vi "Configure Over Voltage Limit.vi"(8 "error in (no error)":errorcluster, 10 "Over Voltage Setting":T1, 11 "BK-Precision in":refnum<class "BK-Precision.lvclass">) -> (0 "error out":errorcluster, 3 "BK-Precision out":refnum<class "BK-Precision.lvclass">)   [LabVIEW 2021, in "DC PWS.lvlib" / "BK-Precision.lvclass"]
uses:
  BK-Precision.lvclass
  BK-Precision.lvclass/BK-Precision.ctl
  <instrlib>/BK Precision 911X Series/BK Precision 911X Series.lvlib
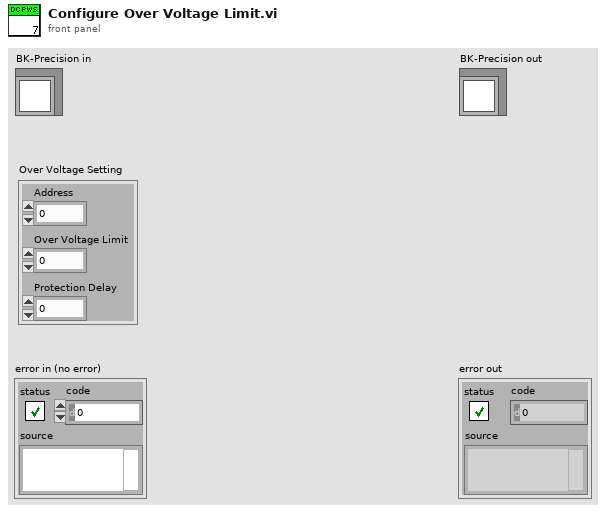
[diagram p1: front panel]
types:
  T1 = cluster{"Address":dbl, "Over Voltage Limit":dbl, "Protection Delay":dbl}
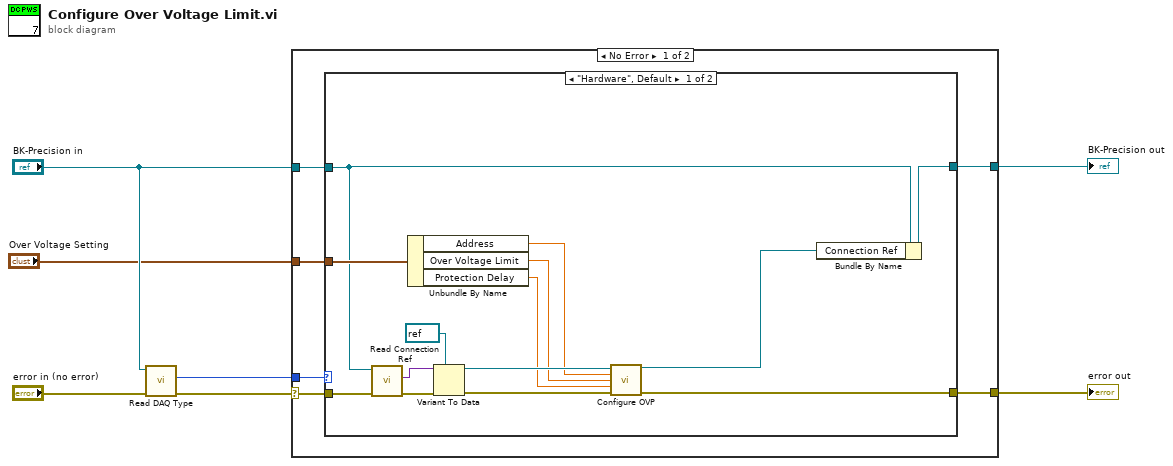
[diagram p0: block diagram]
diagram:
  n1 = call "Read DAQ Type.vi"("error in (no error)"="error in (no error)", "BK-Precision in"="BK-Precision in") -> ("error out"=w6:errorcluster, "Type"=w5:enum16{"Hardware", "Simulation"})  [unwired: 7 in, 1 out]
  n2 = case shown="No Error" w6 {
    selector: w6 -> [w13 w30]
    tunnel: w5 -> [w12 _]
    tunnel: "BK-Precision in" -> [w11 w31]
    tunnel: "Over Voltage Setting" -> [w10 _]
    tunnel: [w9 w31] -> w2
    tunnel: [w8 w30] -> w1
    frame No Error {
      n3 = case shown="\"Hardware\", Default" w12 {
        tunnel: w13 -> [w27 w28]
        tunnel: w11 -> [w17 w29]
        tunnel: w10 -> [w21 _]
        tunnel: [w15 w29] -> w9
        tunnel: [w16 w28] -> w8
        frame "Hardware", Default {
          n4 = call "Read Connection Ref.vi"("error in (no error)"=w27, "BK-Precision in"=w17) -> ("error out"=w26:errorcluster, "Conn Ref"=w25:variant)  [unwired: 7 in, 1 out]
          n5 = Unbundle By Name(w21) -> ("Address"=w18:dbl, "Over Voltage Limit"=w19:dbl, "Protection Delay"=w20:dbl)
          n6 = Variant To Data(error in=w26, type=refnum<visa-resource-name> refnum ("VISA resource name"), Variant=w25) -> (data=w22:refnum<visa-resource-name>, error out=w23:errorcluster)
          n7 = call <instrlib>:"Configure OVP.vi"("VISA resource name"=w22, "Address (0)"=w18, "Voltage Limit (80.000 V)"=w19, "Protection Delay (0.001)"=w20, "error in (no error)"=w23) -> ("VISA resource name out"=w14:refnum<visa-resource-name>, "error out"=w16:errorcluster)  [unwired: 9 in]
          n8 = Bundle By Name(cluster=w17, "Connection Ref"=w14) -> (w15:refnum<class "BK-Precision.lvclass">)
        }
        frame "Simulation" {
        }
      }
    }
    frame Error {
    }
  }
  "error out" <- w1
  "BK-Precision out" <- w2
